vi "GetReportPath.vi"(8 "error in (no error)":errorcluster, 11 "default path":path) -> (0 "error out":errorcluster, 3 "ReportPath":path)   [LabVIEW 2014]
uses:
  <vilib>/Utility/config.llb/Read Key (Path).vi
  <vilib>/Utility/config.llb/NI_LVConfig.lvlib
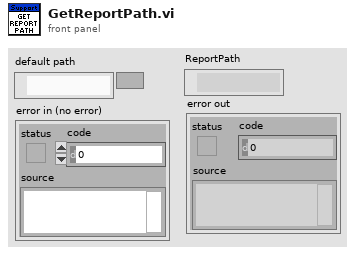
[diagram p1: front panel]
types:
  T1 = typedef "NI_LVConfig.lvlib/Config Data RefNum.ctl" = refnum<k1>
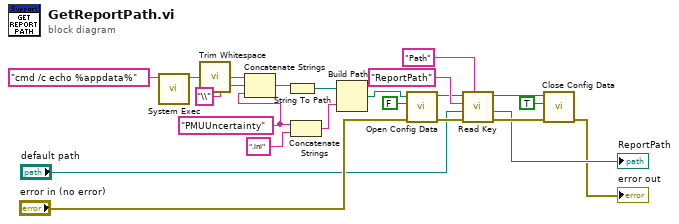
[diagram p0: block diagram]
diagram:
  w19 = "PMUUncertainty" ("string")
  n1 = call <vilib>:"System Exec.vi"("command line"="cmd /c echo %appdata%") -> ("standard output"=w15:string)  [unwired: 7 in, 3 out]
  n2 = call <vilib>:"Trim Whitespace.vi"("string"=w15) -> ("trimmed string"=w14:string)  [unwired: 1 in]
  n3 = Concatenate Strings(w14, "\\" ("string"), w19) -> (w21:string)
  n4 = String To Path(string=w21) -> (path=w20:path)
  n5 = Concatenate Strings(w19, ".ini" ("string")) -> (w17:string)
  n6 = Build Path(base path=w20, name or relative path=w17) -> (appended path=w12:path)
  n7 = call <vilib>:"Open Config Data.vi"("error in (no error)"="error in (no error)", "create file if necessary (T)"=FALSE, "configuration file path"=w12) -> ("error out"=w10:errorcluster, "refnum"=w7:T1)  [unwired: 6 in, 1 out]
  n8 = call-poly <vilib>:"Read Key.vi"("section"="Path", "error in (no error)"=w10, "default value"="default path", "key"="ReportPath", "refnum"=w7) -> ("error out"=w3:errorcluster, "value"=→"ReportPath":path, "refnum out"=w5:T1)  [unwired: 3 in, 1 out]
  n9 = call <vilib>:"Close Config Data.vi"("error in (no error)"=w3, "write file if changed (T)"=TRUE, "refnum"=w5) -> ("error out"=→"error out":errorcluster)  [unwired: 7 in, 1 out]
